vi "Is Indicator.vi"(11 "Control in":refnum<class "Control.lvclass">) -> (2 "Indicator":bool)   [LabVIEW 2020, in "VolatusGUI.lvlib" / "Control.lvclass"]
uses:
  Control.lvclass
  Control.lvclass/Control.ctl
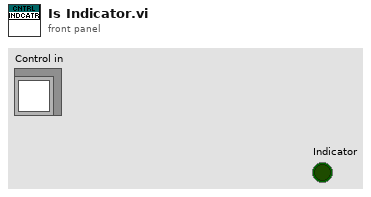
[diagram p1: front panel]
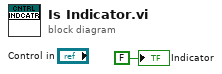
[diagram p0: block diagram]
diagram:
  "Indicator" <- FALSE ("Indicator")
